vi "Desired Position.vi"() -> ()   [LabVIEW 2020]
panel:
  out "Servo Position":dbl
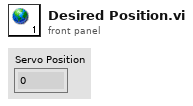
[diagram p1: front panel]
diagram:
